vi "CThread VI Reference.vi"   [LabVIEW 2012, in "CThread.lvlib"]
uses:
  CThread.lvlib
  XNodes/referencenode/CThread VI Reference.xnode
  Base/CThread Base - VI Reference.vi
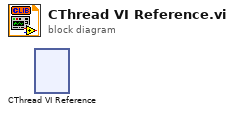
[diagram p0: block diagram]
diagram:
  n1 = xnode "CThread VI Reference"() -> ()  [unwired: 1 out]
